vi "Fetch Messages.vi"(8 "Error In":errorcluster, 11 "Greetings File Path":path) -> (0 "Error Out":errorcluster, 2 "Greetings":cluster{"Language":string, "Message":string}[](array[cluster]))   [LabVIEW 2014]
doc: "Reads the UTF-8 encoded text file that contains the greetings in the various languages, and outputs its contents in a format compatible with a LabVIEW combo box.\n\nCopyright (c) 2019 Sze Howe Koh.\nThis code is licensed under the MIT license."
uses:
  <vilib>/Utility/config.llb/Read Key (String).vi
  <vilib>/Utility/config.llb/NI_LVConfig.lvlib
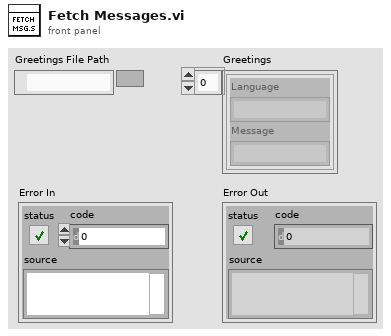
[diagram p1: front panel]
types:
  T1 = typedef "NI_LVConfig.lvlib/Config Data RefNum.ctl" = refnum<k1>
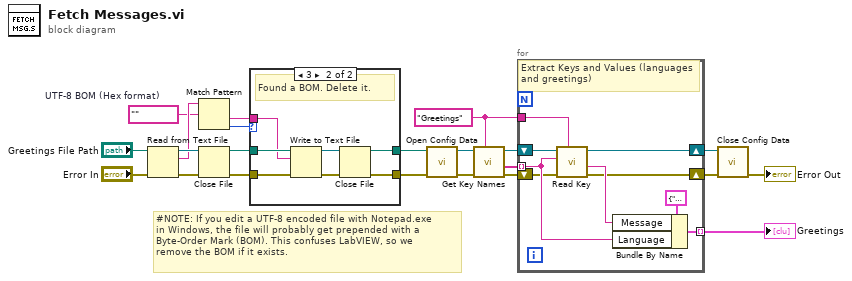
[diagram p0: block diagram]
diagram:
  w8 = "﻿"  # UTF-8 BOM (Hex format)
  w20 = "Greetings" ("section")
  # "#NOTE: If you edit a UTF-8 encoded file with Notepad.exe\nin Windows, the file will probably get prepended with a\nByte-Order Mark (BOM). This confuses LabVIEW, so we\nremove the BOM if it exists."
  n1 = Read from Text File(file (use dialog)="Greetings File Path", error in="Error In") -> (refnum out=w10:refnum<file>, text=w9:string, error out=w3:errorcluster)  [unwired: 2 in, 1 out]
  n2 = Match Pattern(string=w9, regular expression=w8) -> (after substring=w6:string, offset past match=w7:i32)  [unwired: 1 in, 2 out]
  n3 = Close File(refnum=w10, error in=w3) -> (path=w5:path, error out=w2:errorcluster)
  n4 = case shown="3" w7 {
    tunnel: w6 -> [_ w30]
    tunnel: w5 -> [w24 w31]
    tunnel: [w24 w28] -> w4
    tunnel: w2 -> [w23 w27]
    tunnel: [w23 w25] -> w1
    frame Default {
      # "No BOM, all good."
    }
    frame 3 {
      # "Found a BOM. Delete it."
      n5 = Write to Text File(file (use dialog)=w31, text=w30, error in=w27) -> (refnum out=w29:refnum<file>, error out=w26:errorcluster)  [unwired: 1 in, 1 out]
      n6 = Close File(refnum=w29, error in=w26) -> (path=w28:path, error out=w25:errorcluster)
    }
  }
  n7 = call <vilib>:"Open Config Data.vi"("error in (no error)"=w1, "configuration file path"=w4) -> ("error out"=w17:errorcluster, "refnum"=w19:T1)  [unwired: 7 in, 1 out]
  n8 = call <vilib>:"Get Key Names.vi"("section"=w20, "error in (no error)"=w17, "refnum"=w19) -> ("error out"=w16:errorcluster, "key names"=w21:string[], "refnum out"=w18:T1)  [unwired: 5 in, 1 out]
  n9 = for {
    tunnel: w20 -> [w39]
    shift-right: [w38] -> w22
    shift-left: w18 -> [w40]
    tunnel: w21 -> [w37] mode=indexing
    tunnel: [w36] -> w14 mode=indexing
    shift-right: [w32] -> w15
    shift-left: w16 -> [w33]
    # "Extract Keys and Values (languages and greetings)"
    n10 = call-poly <vilib>:"Read Key.vi"("section"=w39, "error in (no error)"=w33, "key"=w37, "refnum"=w40) -> ("error out"=w32:errorcluster, "value"=w34:string, "refnum out"=w38:T1)  [unwired: 4 in, 1 out]
    n11 = Bundle By Name(cluster=cluster{"Language":string, "Message":string} {"Language"="", "Message"=""}, "Message"=w34, "Language"=w37) -> (w36:cluster{"Language":string, "Message":string})
  }
  "Greetings" <- w14
  n12 = call <vilib>:"Close Config Data.vi"("error in (no error)"=w15, "refnum"=w22) -> ("error out"=→"Error Out":errorcluster)  [unwired: 8 in, 1 out]
